vi "Update_xPos.vi"(7 "FastUpdateAxis":i32=1, 8 "error in (no error)":errorcluster, 11 "VISA resource name":refnum<visa-resource-name>) -> (0 "error out":errorcluster, 1 "x_Moving":bool, 2 "x_pos":dbl, 3 "tickcount_pos":u32)   [LabVIEW 2012, in "ESP300.lvlib"]
doc: "Performs an instrument error query before terminating the software connection to the instrument."
uses:
  <instrlib>/ESP300/ESP300.lvlib
  <instrlib>/ESP300/Public/Position_ESP300.vi
panel:
  out "iter.":i32
  out "Read Buffer":string
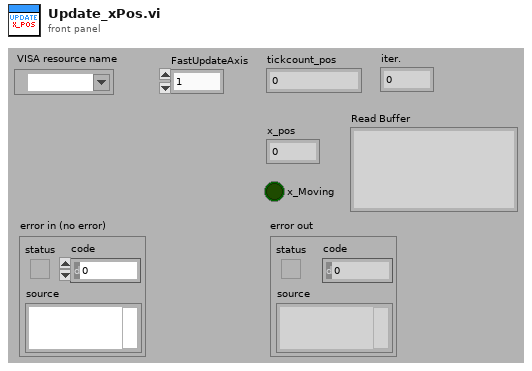
[diagram p1: front panel]
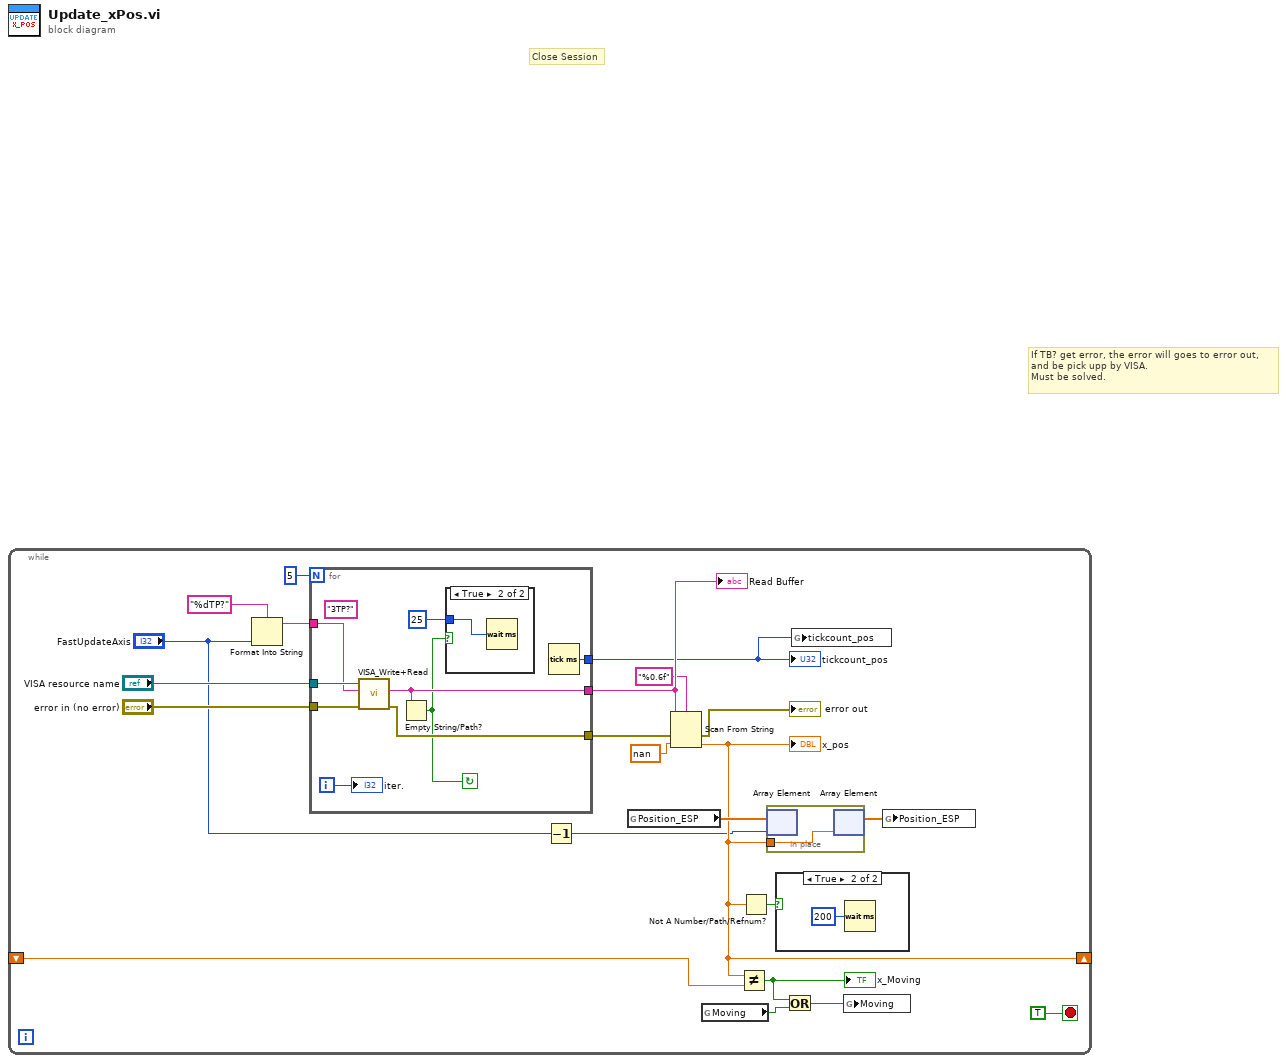
[diagram p0: block diagram]
diagram:
  # "If TB? get error, the error will goes to error out, \nand be pick upp by VISA.\nMust be solved."
  # "Close Session"
  n1 = while {
    shift-right: [w6] -> _
    shift-left: _ -> [w15]
    stop <- TRUE stop-if-true
    n2 = Format Into String(format string="%dTP?" ("initial string"), "FastUpdateAxis") -> (resulting string=w4:string)  [unwired: 2 in, 1 out]
    n3 = for {
      N: 5 -> [_]
      tunnel: "VISA resource name" -> [w31]
      tunnel: [w27] -> w21
      tunnel: "error in (no error)" -> [w30]
      tunnel: [w29] -> w17
      tunnel: [w28] -> w11
      tunnel: w4 -> [w23]
      i -> [w24]
      stop <- w26 continue-if-true
      (unwired) "3TP?" ("string")
      n4 = call <instrlib>:"VISA_Write+Read.vi"("error in (no error)"=w30, "Write Buffer"=w23, "VISA resource name"=w31) -> ("error out"=w29:errorcluster, "readout"=w27:string)  [unwired: 6 in, 1 out]
      n5 = Empty String/Path?(string/path=w27) -> (empty?=w26:bool)
      n6 = case shown="True" w26 {
        tunnel: u32 25 ("milliseconds to wait") -> [_ w32]
        frame False {
        }
        frame True {
          n7 = Wait (ms)(milliseconds to wait=w32) -> ()  [unwired: 1 out]
        }
      }
      n8 = Tick Count (ms)() -> (millisecond timer value=w28:u32)
      "iter." <- w24
    }
    "tickcount_pos" <- w11
    "Read Buffer" <- w21
    n9 = Decrement(x="FastUpdateAxis") -> (x-1=w1:i32)
    n10 = global read "Position_ESP300.vi" "Position_ESP"() -> (w13:dbl[])
    n11 = Scan From String(format string="%0.6f", input string=w21, error in=w17, default 1=nan ("default value 1")) -> (error out=→"error out":errorcluster, output 1=w6:dbl)  [unwired: 1 in, 2 out]
    "x_pos" <- w6
    n12 = global read "Position_ESP300.vi" "Moving"() -> (w9:bool)
    n13 = Not Equal?(x=w6, y=w15) -> (x != y?=w8:bool)
    "x_Moving" <- w8
    n14 = Not A Number/Path/Refnum?(number/path/refnum=w6) -> (NaN/Path/Refnum?=w16:bool)
    n15 = in-place {
      in-place-border: w6 -> [w33]
      n16 = in-place-array #1(w13, w1) -> ()  [unwired: 1 out]
      n17 = in-place-array #1(w33) -> (w14:dbl[])  [unwired: 1 out]
    }
    n18 = case shown="True" w16 {
      frame False {
      }
      frame True {
        n19 = Wait (ms)(milliseconds to wait=u32 200) -> ()  [unwired: 1 out]
      }
    }
    n20 = Or(x=w8, y=w9) -> (x .or. y?=w10:bool)
    n21 = global write "Position_ESP300.vi" "tickcount_pos"(w11) -> ()
    n22 = global write "Position_ESP300.vi" "Moving"(w10) -> ()
    n23 = global write "Position_ESP300.vi" "Position_ESP"(w14) -> ()
  }
